vi "TestVision.vi"() -> ()   [LabVIEW 2019]
uses:
  <vilib>/userDefined/High Color/IMAQdx.ctl
  <vilib>/vision/driver/NI_Vision_Acquisition_Software.lvlib
  <vilib>/vision/NI_Vision_Development_Module.lvlib
panel:
  in  "ROI Descriptor":T1 {"Contours"."Type" items=["No Selection", "Point", "Line", "Rectangle", "Oval", "Polygon", "Free", "Annulus", "Unused2", "Unused3", "Broken Line", "Free Hand Line", "Rotated Rectangle"]}
  out "Fitted Circle":T2 {"Average SNR (dB)" format="%.2f"; "Average Strength" format="%.2f"; "Roundness (Real-World)" format="%.2f"; "Radius (Real-World)" format="%.2f"; "Center (Real-World)"."Y" format="%.2f"; "Center (Real-World)"."X" format="%.2f"; "Radius (Pixels)" format="%.2f"; "Center (Pixels)"."Y" format="%.2f"; "Center (Pixels)"."X" format="%.2f"}
  out "Circle Found":bool
  in  "stop":bool
  out "Image 2":T3(plugin-control)
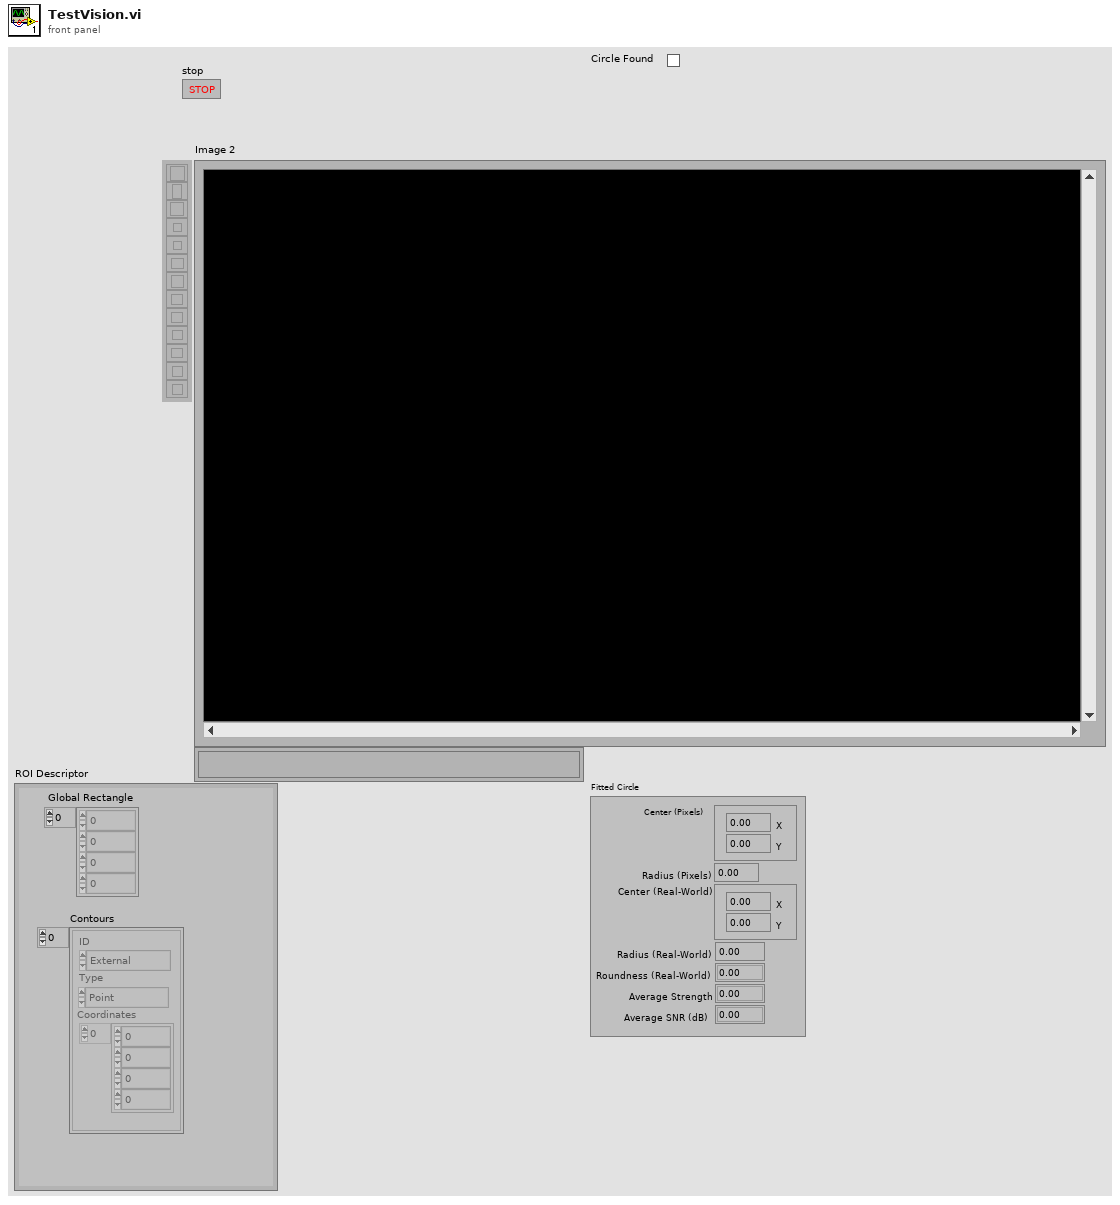
[diagram p1: front panel]
types:
  T1 = cluster{"Global Rectangle":i32[], "Contours":cluster{"ID":enum32{"External", "Internal"}, "Type":u32, "Coordinates":i32[]}[]}
  T2 = cluster{"Center (Pixels)":cluster{"X":sgl, "Y":sgl}, "Radius (Pixels)":dbl, "Center (Real-World)":cluster{"X":sgl, "Y":sgl}, "Radius (Real-World)":dbl, "Roundness (Real-World)":dbl, "Average Strength":dbl, "Average SNR (dB)":dbl}
  T3 = typedef "IMAQ Image.ctl" = refnum<image>
  T4 = typedef "IMAQdx.ctl" = refnum<k21>
  T5 = cluster{"Process":enum16{"Get First Edge", "Get First + Last Edge", "Get All Edges", "Get Best Edge"}, "Step Size":dbl, "Max Pixel Radius":i32}
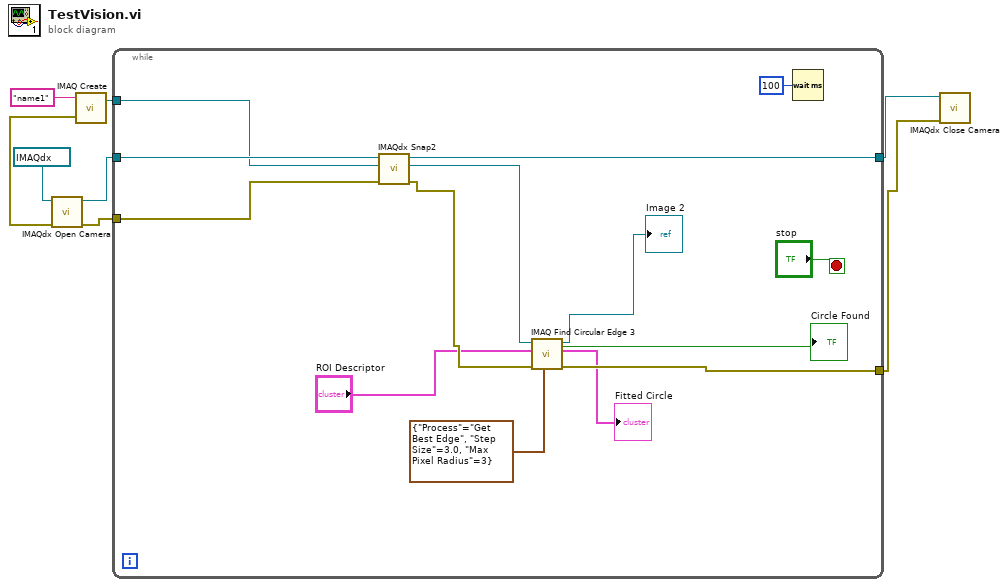
[diagram p0: block diagram]
diagram:
  n1 = call "IMAQ Create"("Image Name"="name1") -> ("New Image"=w3:T3, "error out"=w1:errorcluster)  [unwired: 4 in]
  n2 = call <vilib>:"IMAQdx Open Camera.vi"("error in"=w1, "Session In"=T4 "cam0") -> ("error out"=w6:errorcluster, "Session Out"=w5:T4)  [unwired: 8 in]
  n3 = while {
    tunnel: [w22] -> w8
    tunnel: w6 -> [w21]
    tunnel: w5 -> [w20]
    tunnel: w3 -> [w19]
    tunnel: [w13] -> w2
    stop <- "stop" stop-if-true
    n4 = call <vilib>:"IMAQdx Snap2.vi"("error in"=w21, "Image In"=w19, "Session In"=w20) -> ("error out"=w16:errorcluster, "Image Out"=w15:T3, "Session Out"=w22:T4)  [unwired: 6 in]
    n5 = call "IMAQ Find Circular Edge 3"("Circle Fit Options"=T5 {"Process"=enum."Get Best Edge", "Step Size"=3.0, "Max Pixel Radius"=3}, "error in (no error)"=w16, "ROI Descriptor"="ROI Descriptor", "Image"=w15) -> ("error out"=w13:errorcluster, "Fitted Circle"=→"Fitted Circle":T2, "Image Out"=→"Image 2":T3, "Circle Found"=→"Circle Found":bool)  [unwired: 3 in, 1 out]
    n6 = Wait (ms)(milliseconds to wait=u32 100) -> ()  [unwired: 1 out]
  }
  n7 = call <vilib>:"IMAQdx Close Camera.vi"("error in"=w2, "Session In"=w8) -> ()  [unwired: 9 in, 1 out]
